vi "Filter.vi"() -> ()   [LabVIEW 2022 SP3]
uses:
  Control 1.ctl
  <vilib>/Platform/TimedLoop/XDataNode/timing_clust.ctl
  <vilib>/Platform/TimedLoop/XDataNode/nitl_modes.ctl
  <vilib>/Platform/TimedLoop/XDataNode/wakeup.ctl
  <vilib>/rvi/FXPMathLib/FxpConvert/subVIs/nifxpmath_Convert_SimConfig.ctl
  <vilib>/fxp/LVFixedPointQuantizationPolicyTypeDef.ctl
  <vilib>/fxp/LVFixedPointOverflowPolicyTypeDef.ctl
  <vilib>/rvi/FXPMathLib/basic elements/DSP48E/simVIs/niFpgaDsp48eSimulationState.ctl
  <vilib>/rvi/FXPMathLib/basic elements/DSP48E/subVIs/niFpgaDsp48eType.ctl
  <vilib>/rvi/FXPMathLib/basic elements/DSP48E/subVIs/niFpgaDsp48eAlumodeOpmodeCarryinselState.ctl
  <vilib>/rvi/FXPMathLib/basic elements/DSP48E/subVIs/niFpgaDsp48eUseMultiplierState.ctl
  <vilib>/rvi/FXPMathLib/basic elements/DSP48E/subVIs/niFpgaDsp48eLogicUnitModeState.ctl
  <vilib>/rvi/FXPMathLib/basic elements/DSP48E/subVIs/niFpgaDsp48eSelectPatternState.ctl
  <vilib>/rvi/FXPMathLib/basic elements/DSP48E/subVIs/niFpgaDsp48eSelectMaskState.ctl
  <vilib>/rvi/FXPMathLib/basic elements/DSP48E/subVIs/niFpgaDsp48eAutoresetState.ctl
  <vilib>/rvi/FXPMathLib/basic elements/DSP48E/simVIs/niFpgaDsp48eResets.ctl
  <vilib>/rvi/FXPMathLib/basic elements/DSP48E/simVIs/niFpgaDsp48eEnables.ctl
  <vilib>/rvi/FXPMathLib/basic elements/DSP48E/simVIs/niFpgaDsp48eRegisters.ctl
  <vilib>/rvi/FXPMathLib/FxpSinAndCos/subVIs/nifxpmath_SinAndCos_SimConfig.ctl
  <vilib>/rvi/Emulation/niFpgaSctlEmulationGetInTimedLoop.vi
  <vilib>/rvi/Emulation/niFpgaEmulationReportErrorSimple.vi
  <vilib>/rvi/Emulation/niFpgaGetClockAttributes.vi
  <vilib>/rvi/Emulation/niFpgaCriticalErrorInLSC.vi
  <vilib>/rvi/eio/common/nirviEmuTemplateMethod_errors.vi
  <vilib>/rvi/FXPMathLib/FxpConvert/simVIs/DllFxpConvertTemp_sub.vi
  <vilib>/rvi/FXPMathLib/basic elements/DSP48E/simVIs/niFpgaDsp48eCheckMode.vi
  <vilib>/rvi/FXPMathLib/basic elements/DSP48E/simVIs/niFpgaDsp48eReportInvalidMode.vi
  <vilib>/rvi/FXPMathLib/basic elements/DSP48E/simVIs/niFpgaDsp48eSimMultiplier.vi
  <vilib>/rvi/FXPMathLib/basic elements/DSP48E/simVIs/niFpgaDsp48eSimArithmetic.vi
  <vilib>/rvi/FXPMathLib/basic elements/DSP48E/simVIs/niFpgaDsp48eSimPatternDetect.vi
  <vilib>/rvi/FXPMathLib/basic elements/DSP48E/simVIs/niFpgaDsp48eSimP.vi
  <vilib>/rvi/FXPMathLib/basic elements/DSP48E/simVIs/niFpgaDsp48eSimUpdateState.vi
  <vilib>/rvi/FXPMathLib/FxpSinAndCos/simVIs/DllFxpSinAndCosTemp_sub.vi
  <vilib>/rvi/DataTransferAndStorage/Container/Common/niFpgaContainerExecOnDevCompGetState.vi
  <vilib>/rvi/Emulation/niFpgaEmulationIsFPGAContextNoSignature.vi
  <vilib>/rvi/errors/niFpgaSetErrorForExecOnDevCompSimple.vi
  <vilib>/rvi/eio/common/nirviEmuReportErrorAndStop.vi
  <vilib>/rvi/DataTransferAndStorage/Container/Common/niFpgaContainerGetUniqueNameForEmu.vi
  <vilib>/rvi/FIFO/Fifo_Resource/nirvififoEmulationSetSize.vi
  <vilib>/rvi/FIFO/Fifo_Resource/nirviFifoEmulationQueueMgr.vi
  <instcachedir>/0/nirviFifoEmulationQueueMgr_E5CAEC123FF24DC58D834DCA3CDAA9B5.lvgen/nirviFifoEmulationQueueMgr_E5CAEC123FF24DC58D834DCA3CDAA9B5_032.vi
  <vilib>/rvi/FIFO/Fifo_Resource/nirvififoEmulationDetermineInputValidOut.vi
  <vilib>/rvi/FIFO/Fifo_Resource/nirvififoEmulationCreateLock.vi
  <vilib>/rvi/Emulation/niFpgaProcessEmulError.vi
  <vilib>/rvi/FIFO/Fifo_Resource/nirvififoEmulationObtainLock.vi
  <vilib>/rvi/FIFO/Fifo_Resource/nirvififoEmulationReleaseLock.vi
  <vilib>/rvi/occurrence/nirviWaitOnOccurrenceBase.vi
  <vilib>/rvi/errors/nirviReportUnexpectedCaseInternalError.vi
  <vilib>/rvi/errors/nirviReportUnexpectedCaseInternalError (U32).vi
  <vilib>/Utility/error.llb/Clear Errors.vi
  <vilib>/rvi/interface/RandomDataEmulation/niFpgaRandomDataHandleErrors.vi
  <instcachedir>/0/nirviFifoEmulationQueueMgr_E5CAEC123FF24DC58D834DCA3CDAA9B5.lvgen/nirviFifoEmulationQueueMgr_E5CAEC123FF24DC58D834DCA3CDAA9B5_039.vi
  <instcachedir>/0/nirviFifoEmulationQueueMgr_E5CAEC123FF24DC58D834DCA3CDAA9B5.lvgen/nirviFifoEmulationQueueMgr_E5CAEC123FF24DC58D834DCA3CDAA9B5_034.vi
  <vilib>/platform/TimedLoop/XDataNode/XDataNode.xnode
  <vilib>/eio/EIONode/EIONode.xnode
  <vilib>/rvi/FXPMathLib/FxpConvert/XNode/nifxpmath_Convert.xnode
  <vilib>/rvi/FXPMathLib/basic elements/DSP48E/XNode/niFpgaDsp48e.xnode
  <vilib>/rvi/FXPMathLib/FxpAdd/XNode/nifxpmath_Add.xnode
  <vilib>/rvi/FXPMathLib/FxpSinAndCos/XNode/nifxpmath_SinAndCos.xnode
  <vilib>/rvi/DataTransferAndStorage/Container/XNode/niFpgaContainer.xnode
  <vilib>/rvi/FIFO/Fifo_Resource/niFpgaFifoEmulationRefIn.vi
  <vilib>/Platform/TimedLoop/XDataNode/XDNodeRunTimeDep.lvlib
  <vilib>/rvi/FXPMathLib/sim/FxpSim.dll
panel:
  out "x":fxp<+/-,25,2>
  in  "White Noise\nAmplitude":u16=5000
  in  "Sine\ndelta_t":fxp<+/-,64,4>
  in  "Add white noise?":bool
  out "y":fxp<+/-,25,2>
  in  "Signal Generator\nSelect":T1
  in  "DMA FIFO Resolution":u32
  in  "Square Frequency":i16
  in  "Sawtooth Frequency":i16
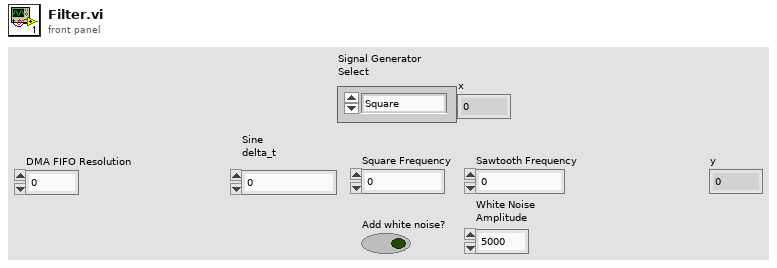
[diagram p1: front panel]
types:
  T1 = typedef "Control 1.ctl" = enum16{"Square", "Sawtooth", "Sine"}
  T2 = typedef "XDNodeRunTimeDep.lvlib/timing_clust.ctl" = cluster{"Expected End [f-1]":u64, "Actual End [f-1]":u64, "Finished Late? [f-1]":bool, "Expected End [i-1]":u64, "Actual End [i-1]":u64, "Finished Late? [i-1]":bool, "Expected Start [i]":u64, "Actual Start [i]":u64, "Expected Start [f]":u64, "Actual Start [f]":u64, "Source Name":string, "Structure Name":string, "Period":i64, "Deadline":i64, "Offset":i64, "Start":i64, "Priority":i32, "Timeout":i32, "Mode":T3, "Wakeup Reason":T4, "Error":errorcluster, "Source Type":string, "Secondary Source Type":string, "Global End Time":u64, "Global Start Time":u64, "Frame Duration":u64, "Iteration Duration":u64, "Assigned CPU":i32, "I/O Scan Engine Mode":u32}
  T3 = typedef "XDNodeRunTimeDep.lvlib/nitl_modes.ctl" = enum32{"No Change", "Process missed periods, maintain original phase", "Discard missed periods, maintain original phase", "Process missed periods, ignore original phase", "Discard missed periods, ignore original phase"}
  T4 = typedef "XDNodeRunTimeDep.lvlib/wakeup.ctl" = enum32{"Normal", "Aborted", "Asynchronous wakeup", "Timing source error", "Timed loop error", "Timeout"}
  T5 = typedef "niFpgaDsp48eRegisters.ctl" = cluster{"a register 1":fxp<+/-,30,30>, "a register 2":fxp<+/-,30,30>, "b register 1":fxp<+/-,18,18>, "b register 2":fxp<+/-,18,18>, "c register":fxp<+/-,48,48>, "d register":fxp<+/-,25,25>, "ad register":fxp<+/-,27,27>, "m register":fxp<+/-,45,45>, "opmode register":fxp<+,7,7>, "alumode register":fxp<+,4,4>, "carryinsel register":fxp<+,3,3>, "inmode register":fxp<+,5,5>, "carryin register":bool, "multcarryin register":bool, "p registers":fxp<+/-,48,48>, "carryout register":fxp<+,4,4>, "carrycascout register":bool, "multsignout register":bool, "patterndetect register":bool, "patternbdetect register":bool, "patterndetect register 2":bool, "patternbdetect register 2":bool}
  T6 = typedef "niFpgaDsp48eEnables.ctl" = cluster{"cea1":bool, "cea2":bool, "cead":bool, "cealumode":bool, "ceb1":bool, "ceb2":bool, "cec":bool, "cecarryin":bool, "cectrl":bool, "ced":bool, "ceinmode":bool, "cem":bool, "cemultcarryin":bool, "cep":bool}
  T7 = typedef "niFpgaDsp48eResets.ctl" = cluster{"rsta":bool, "rstallcarryin":bool, "rstalumode":bool, "rstb":bool, "rstc":bool, "rstctrl":bool, "rstd":bool, "rstinmode":bool, "rstm":bool, "rstp":bool}
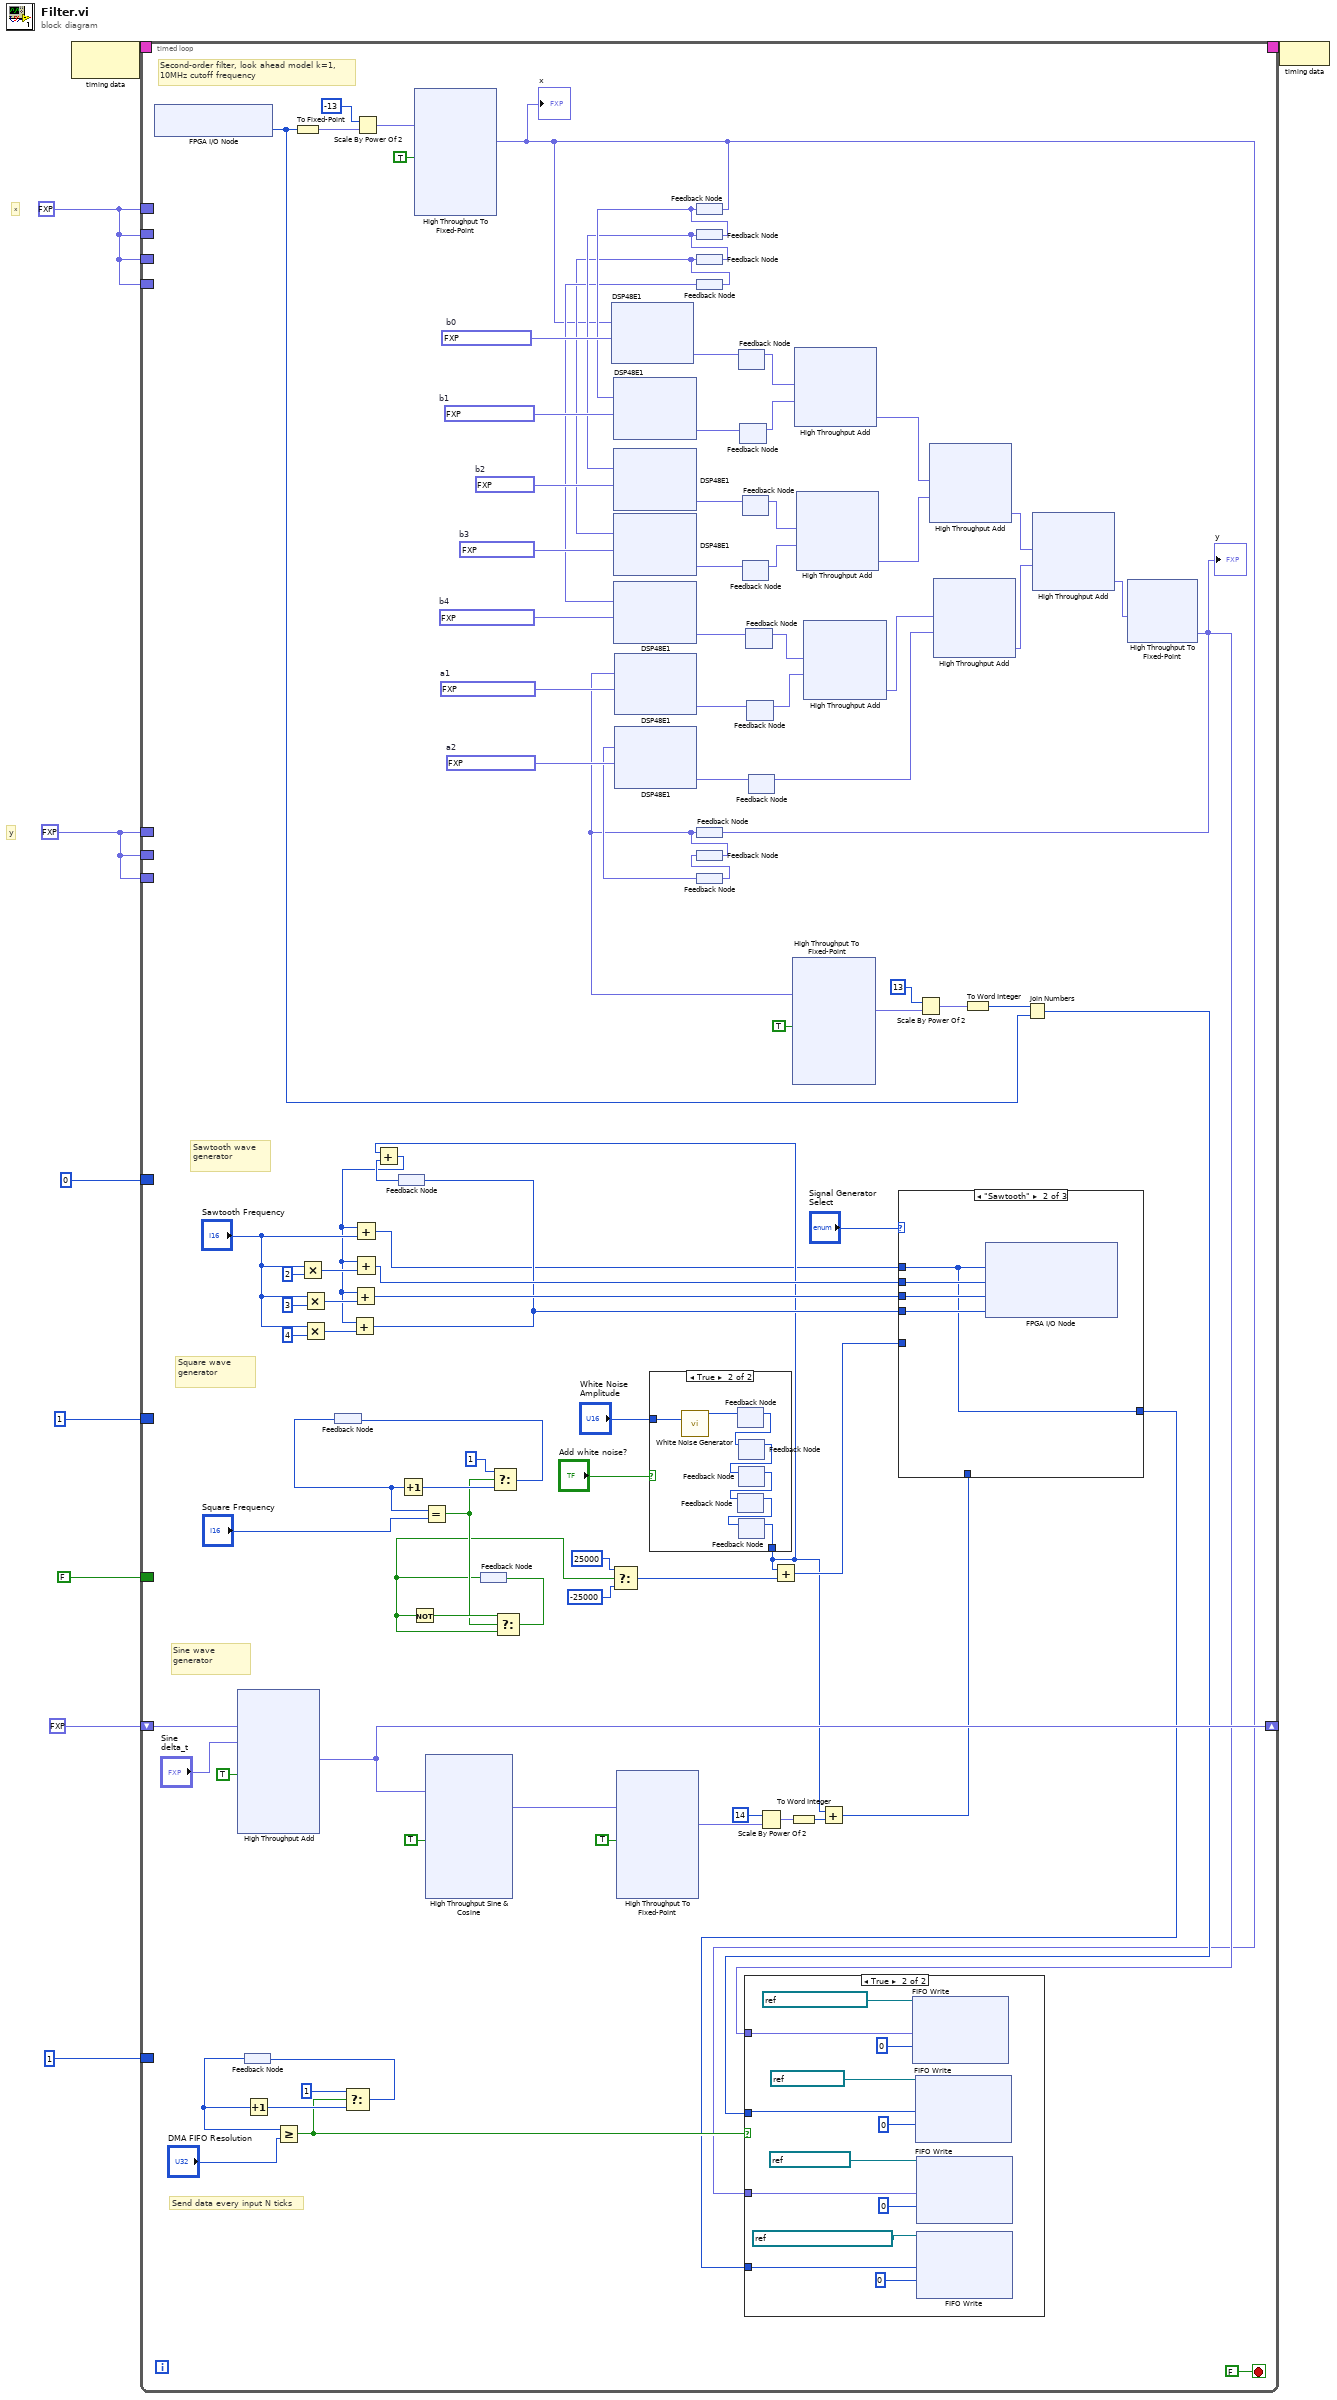
[diagram p0: block diagram]
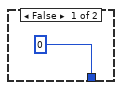
[diagram p2: hidden frame]
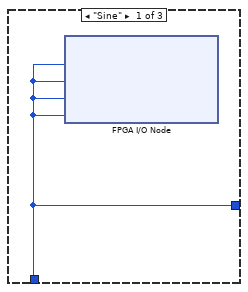
[diagram p4: hidden frame]
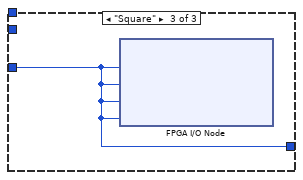
[diagram p5: hidden frame]
diagram:
  w2 = fxp<+/-,25,2> 0.0 ("x+y")
  w3 = fxp<+/-,25,2> 0.0 ("x+y")
  # "x"
  # "y"
  n1 = node-c288() -> (w9:T2)  [unwired: 1 in]
  n2 = timed-loop {
    timing: w9 -> [_]
    timing-out: [_] -> w8
    border: i16 1 ("Timeout") -> [_]
    border: i16 0 ("Timeout") -> [_]
    border: FALSE -> [_]
    border: u32 1 ("Timeout") -> [_]
    shift-right: [w41] -> _
    shift-left: fxp<+/-,64,4> 0.0 ("Timeout") -> [w43]
    border: w2 -> [_]
    border: w2 -> [_]
    border: w2 -> [_]
    border: w2 -> [_]
    border: w3 -> [_]
    border: w3 -> [_]
    border: w3 -> [_]
    stop <- FALSE stop-if-true
    w69 = fxp<+/-,18,2> 0.0226898193359375  # b4
    w70 = fxp<+/-,18,2> 0.105712890625  # b3
    w72 = fxp<+/-,18,2> -0.24188232421875  # a2
    w73 = fxp<+/-,18,2> 0.7253570556640625  # a1
    w75 = fxp<+/-,18,2> 0.189453125  # b2
    w76 = fxp<+/-,18,2> 0.152557373046875  # b1
    w77 = fxp<+/-,18,2> 0.046112060546875  # b0
    # "Second-order filter, look ahead model k=1,\n10MHz cutoff frequency"
    # "Send data every input N ticks"
    # "Sine wave\ngenerator"
    # "Sawtooth wave generator"
    # "Square wave\ngenerator"
    n3 = xnode "FPGA I/O Node"() -> ("IO Module\\AI 1 N"=w19:i16)  [unwired: 1 in, 1 out]
    n4 = xnode ("High Throughput Add")("x"=w43, "y"="Sine\ndelta_t", "input valid"=TRUE) -> ("x+y"=w41:fxp<+/-,64,4>)  [unwired: 1 in, 2 out]
    n5 = feedback #1() -> (w106:u32)
    n6 = Increment(x=w106) -> (x+1=w105:u32)
    n7 = Greater Or Equal?(x=w106, y="DMA FIFO Resolution") -> (x >= y?=w18:bool)
    n8 = To Fixed-Point(number=w19) -> (fixed-point=w47:fxp<+/-,39,14>)  [unwired: 1 in]
    n9 = Multiply(x="Sawtooth Frequency", y=i16 2) -> (x*y=w93:i16)
    n10 = Multiply(x="Sawtooth Frequency", y=i16 3) -> (x*y=w89:i16)
    n11 = Multiply(x="Sawtooth Frequency", y=i16 4) -> (x*y=w88:i16)
    n12 = feedback #2() -> (w85:i16)
    n13 = Select(t=u32 1, s=w18, f=w105) -> (s? t:f=w103:u32)
    n14 = feedback-in #1(w103) -> ()
    n15 = Scale By Power Of 2(n=i16 -13, x=w47) -> (x*2^n=w46:fxp<+/-,39,14>)
    n16 = feedback #3() -> (w17:i16)
    n17 = Increment(x=w85) -> (x+1=w84:i16)
    n18 = xnode "High Throughput To Fixed-Point"("x"=w46, "input valid"=TRUE) -> ("y"=w10:fxp<+/-,25,2>)  [unwired: 1 in, 2 out]
    "x" <- w10
    n19 = Equal?(x=w85, y="Square Frequency") -> (x = y?=w83:bool)
    n20 = xnode "High Throughput Sine & Cosine"("x (pi)"=w41, "input valid"=TRUE) -> ("sin(x)"=w39:fxp<+/-,16,2>)  [unwired: 1 in, 3 out]
    n21 = feedback #4() -> (w81:bool)
    n22 = Not(x=w81) -> (.not. x?=w97:bool)
    n23 = Select(t=i16 1, s=w83, f=w84) -> (s? t:f=w101:i16)
    n24 = feedback-in #2(w101) -> ()
    n25 = Select(t=w97, s=w83, f=w81) -> (s? t:f=w82:bool)
    n26 = feedback-in #4(w82) -> ()
    n27 = xnode ("DSP48E1")("a"=w10, "b"=w77) -> ("p"=w65:fxp<+/-,48,9>)
    n28 = Select(t=i16 25000 ("y"), s=w81, f=i16 -25000 ("t")) -> (s? t:f=w79:i16)
    n29 = xnode "High Throughput To Fixed-Point"("x"=w39, "input valid"=TRUE) -> ("y"=w36:fxp<+/-,32,16>)  [unwired: 1 in, 2 out]
    n30 = case shown="True" "Add white noise?" {
      tunnel: [i16 0 ("x") w664] -> w16
      tunnel: "White Noise\nAmplitude" -> [_ w661]
      frame False {
      }
      frame True {
        n31 = call "White Noise Generator"("amplitude"=w661) -> ("white noise out"=w662:i16)  [unwired: 14 in]
        n32 = feedback #5() -> (w663:i16)  [unwired: 1 in]
        n33 = feedback-in #5(w662) -> ()
        n34 = feedback #6() -> (w665:i16)  [unwired: 1 in]
        n35 = feedback #7() -> (w667:i16)  [unwired: 1 in]
        n36 = feedback-in #7(w663) -> ()
        n37 = feedback #8() -> (w666:i16)  [unwired: 1 in]
        n38 = feedback-in #6(w666) -> ()
        n39 = feedback-in #8(w667) -> ()
        n40 = feedback #9() -> (w664:i16)  [unwired: 1 in]
        n41 = feedback-in #9(w665) -> ()
      }
    }
    n42 = Add(x=w16, y=w17) -> (x+y=w15:i16)
    n43 = Add(x=w15, y=w88) -> (x+y=w80:i16)
    n44 = Add(x=w15, y=w89) -> (x+y=w99:i16)
    n45 = Add(x=w15, y="Sawtooth Frequency") -> (x+y=w13:i16)
    n46 = Add(x=w15, y=w93) -> (x+y=w100:i16)
    n47 = feedback-in #3(w80) -> ()
    n48 = feedback-in #10(w10) -> ()
    n49 = feedback #10() -> (w74:fxp<+/-,25,2>)
    n50 = xnode ("DSP48E1")("a"=w74, "b"=w76) -> ("p"=w64:fxp<+/-,48,9>)
    n51 = feedback-in #11(w74) -> ()
    n52 = feedback #11() -> (w68:fxp<+/-,25,2>)
    n53 = xnode ("DSP48E1")("a"=w68, "b"=w75) -> ("p"=w63:fxp<+/-,48,9>)
    n54 = feedback-in #12(w68) -> ()
    n55 = feedback #12() -> (w66:fxp<+/-,25,2>)
    n56 = xnode ("DSP48E1")("a"=w66, "b"=w70) -> ("p"=w62:fxp<+/-,48,9>)
    n57 = feedback-in #13(w66) -> ()
    n58 = feedback #13() -> (w67:fxp<+/-,25,2>)
    n59 = xnode ("DSP48E1")("a"=w67, "b"=w69) -> ("p"=w61:fxp<+/-,48,9>)
    n60 = feedback #14() -> (w14:fxp<+/-,25,2>)
    n61 = xnode ("DSP48E1")("a"=w14, "b"=w73) -> ("p"=w30:fxp<+/-,48,9>)
    n62 = feedback-in #15(w14) -> ()
    n63 = feedback #15() -> (w71:fxp<+/-,25,2>)
    n64 = feedback-in #16(w71) -> ()
    n65 = feedback #16() -> (w26:fxp<+/-,25,2>)
    n66 = xnode ("DSP48E1")("a"=w26, "b"=w72) -> ("p"=w29:fxp<+/-,48,9>)
    n67 = feedback-in #17(w65) -> ()
    n68 = feedback #17() -> (w60:fxp<+/-,48,9>)  [unwired: 1 in]
    n69 = feedback #18() -> (w59:fxp<+/-,48,9>)  [unwired: 1 in]
    n70 = feedback-in #18(w64) -> ()
    n71 = feedback #19() -> (w58:fxp<+/-,48,9>)  [unwired: 1 in]
    n72 = feedback-in #19(w63) -> ()
    n73 = feedback #20() -> (w57:fxp<+/-,48,9>)  [unwired: 1 in]
    n74 = feedback-in #20(w62) -> ()
    n75 = feedback #21() -> (w56:fxp<+/-,48,9>)  [unwired: 1 in]
    n76 = feedback-in #21(w61) -> ()
    n77 = feedback #22() -> (w55:fxp<+/-,48,9>)  [unwired: 1 in]
    n78 = feedback-in #22(w30) -> ()
    n79 = feedback #23() -> (w51:fxp<+/-,48,9>)  [unwired: 1 in]
    n80 = feedback-in #23(w29) -> ()
    n81 = Scale By Power Of 2(n=i16 14, x=w36) -> (x*2^n=w35:fxp<+/-,32,16>)
    n82 = Add(x=w16, y=w79) -> (x+y=w27:i16)
    n83 = To Word Integer(number=w35) -> (16bit integer=w34:i16)
    n84 = xnode "High Throughput To Fixed-Point"("x"=w14, "input valid"=TRUE) -> ("y"=w23:fxp<+/-,32,16>)  [unwired: 1 in, 2 out]
    n85 = xnode ("High Throughput Add")("x"=w60, "y"=w59) -> ("x+y"=w54:fxp<+/-,49,10>)
    n86 = xnode ("High Throughput Add")("x"=w58, "y"=w57) -> ("x+y"=w53:fxp<+/-,49,10>)
    n87 = xnode ("High Throughput Add")("x"=w56, "y"=w55) -> ("x+y"=w52:fxp<+/-,49,10>)
    n88 = Add(x=w16, y=w34) -> (x+y=w33:i16)
    n89 = case shown="\"Sawtooth\"" "Signal Generator\nSelect" {
      tunnel: w13 -> [_ w681 _]
      tunnel: w100 -> [_ w684 _]
      tunnel: w99 -> [_ w683 _]
      tunnel: w80 -> [_ w682 _]
      tunnel: w27 -> [_ _ w685]
      tunnel: w33 -> [w680 _ _]
      tunnel: [w680 w681 w685] -> w11
      frame "Sine" {
        n90 = xnode "FPGA I/O Node"("IO Module\\AO 1 N"=w680, "IO Module\\AO 1 N-1"=w680, "IO Module\\AO 1 N-2"=w680, "IO Module\\AO 1 N-3"=w680) -> ()  [unwired: 4 in, 4 out]
      }
      frame "Sawtooth" {
        n91 = xnode "FPGA I/O Node"("IO Module\\AO 1 N"=w681, "IO Module\\AO 1 N-1"=w684, "IO Module\\AO 1 N-2"=w683, "IO Module\\AO 1 N-3"=w682) -> ()  [unwired: 4 in, 4 out]
      }
      frame "Square" {
        n92 = xnode "FPGA I/O Node"("IO Module\\AO 1 N"=w685, "IO Module\\AO 1 N-1"=w685, "IO Module\\AO 1 N-2"=w685, "IO Module\\AO 1 N-3"=w685) -> ()  [unwired: 4 in, 4 out]
      }
    }
    n93 = Scale By Power Of 2(n=i16 13, x=w23) -> (x*2^n=w22:fxp<+/-,32,16>)
    n94 = xnode ("High Throughput Add")("x"=w54, "y"=w53) -> ("x+y"=w50:fxp<+/-,50,11>)
    n95 = xnode ("High Throughput Add")("x"=w52, "y"=w51) -> ("x+y"=w49:fxp<+/-,50,11>)
    n96 = To Word Integer(number=w22) -> (16bit integer=w21:i16)
    n97 = Join Numbers(hi=w21, lo=w19) -> ((hi.lo)=w12:u32)
    n98 = xnode ("High Throughput Add")("x"=w50, "y"=w49) -> ("x+y"=w28:fxp<+/-,51,12>)
    n99 = xnode "High Throughput To Fixed-Point"("x"=w28) -> ("y"=w25:fxp<+/-,25,2>)
    "y" <- w25
    n100 = feedback-in #14(w25) -> ()
    n101 = case shown="True" w18 {
      tunnel: w25 -> [_ w678]
      tunnel: w12 -> [_ w671]
      tunnel: w10 -> [_ w673]
      tunnel: w11 -> [_ w668]
      frame False {
      }
      frame True {
        n102 = xnode ("FIFO Write")("Element"=w678, "Timeout"=0, "FIFO In"=refnum<k21> "Filtered_2_ToHost") -> ()  [unwired: 2 out]
        n103 = xnode ("FIFO Write")("Element"=w671, "Timeout"=0, "FIFO In"=refnum<k21> "XY_ToHost") -> ()  [unwired: 2 out]
        n104 = xnode ("FIFO Write")("Element"=w673, "Timeout"=0, "FIFO In"=refnum<k21> "Raw_ToHost") -> ()  [unwired: 2 out]
        n105 = xnode ("FIFO Write")("Element"=w668, "Timeout"=0, "FIFO In"=refnum<k21> "Generated_Signal_ToHost") -> ()  [unwired: 2 out]
      }
    }
  }
  n106 = node-c288(w8) -> ()
